vi "Read ID.vi"(8 "error in (no error)":errorcluster, 11 "ClassMetadata in":refnum<class "DirectoryMetadata.lvclass">) -> (0 "error out":errorcluster, 2 "ID":string, 3 "ClassMetadata out":refnum<class "DirectoryMetadata.lvclass">)   [LabVIEW 2017, in "DirectoryMetadata.lvclass"]
uses:
  DirectoryMetadata.lvclass
  DirectoryMetadata.lvclass/DirectoryMetadata.ctl
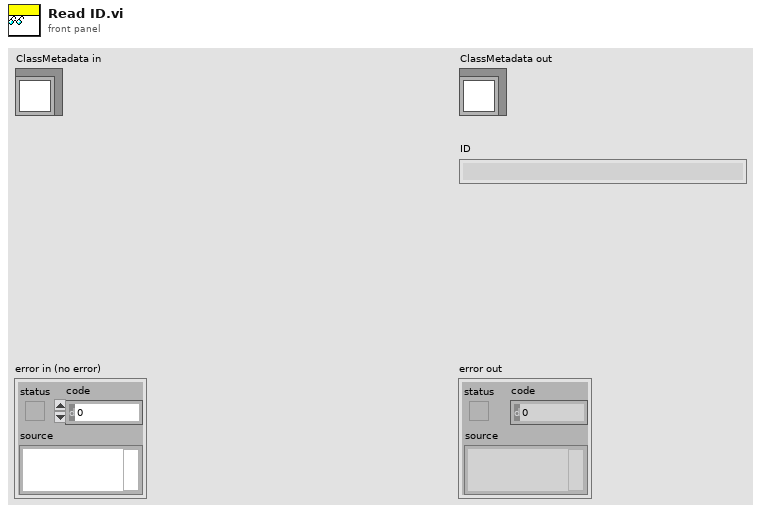
[diagram p1: front panel]
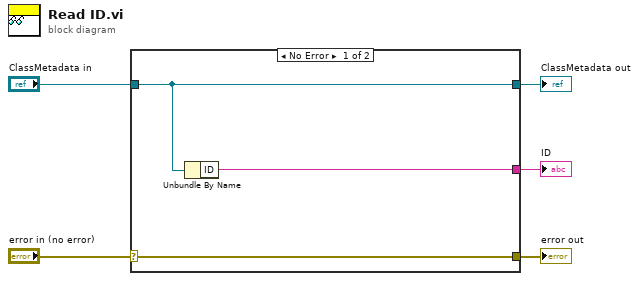
[diagram p0: block diagram]
diagram:
  n1 = case shown="No Error" "error in (no error)" {
    selector: "error in (no error)" -> [w8 w9]
    tunnel: [w8 w9] -> w4
    tunnel: [w7 w10] -> w2
    tunnel: "ClassMetadata in" -> [w7 w10]
    tunnel: [w6 _] -> w1
    frame No Error {
      n2 = Unbundle By Name(w7) -> ("ID"=w6:string)
    }
    frame Error {
    }
  }
  "error out" <- w4
  "ClassMetadata out" <- w2
  "ID" <- w1
